vi "Loop_HW.vi"() -> ()   [LabVIEW 2017, in "WCDrive2018.lvlib"]
uses:
  WCDrive2018.lvlib
  Global_SM Out Data.vi
  Global_HW_Status Out.vi
  ProtoType Code/EXAMPLE 2017 competition code/roboRIO Code/Globals/Global_HW_Address_Assignments.vi
  ENUM_ACT_State.ctl
  ENUM_ACT_Action.ctl
  _SHARE ALL/Global Share All/Global_STOP.vi
  <vilib>/Rock Robotics/WPI/MotorControl/WPI_MotorControlType.ctl
  <vilib>/Rock Robotics/SystemInterfaces/DIO/FPGA_DIOPWMChannel.ctl
  <vilib>/Rock Robotics/WPI/PWM/WPI_PWMDeadband.ctl
  <vilib>/Rock Robotics/SystemInterfaces/DIO/FPGA_DIOChannel.ctl
  <vilib>/Rock Robotics/WPI/MotorControl/WPI_MotorControlDeviceRef.ctl
  <vilib>/Rock Robotics/WPI/RobotDrive/WPI_RobotDriveDevRef.ctl
  Enum_HW Cmd Select.ctl
  Cluster_SM to HW Data.ctl
  570cffa0-ccfc-4d94-993e-2857878fdf6e.vi
panel:
  in  "SM CMD Override":bool
  in  "SM_Cmd":T1
  out "Cycle Time (S)":dbl format="%.3g"
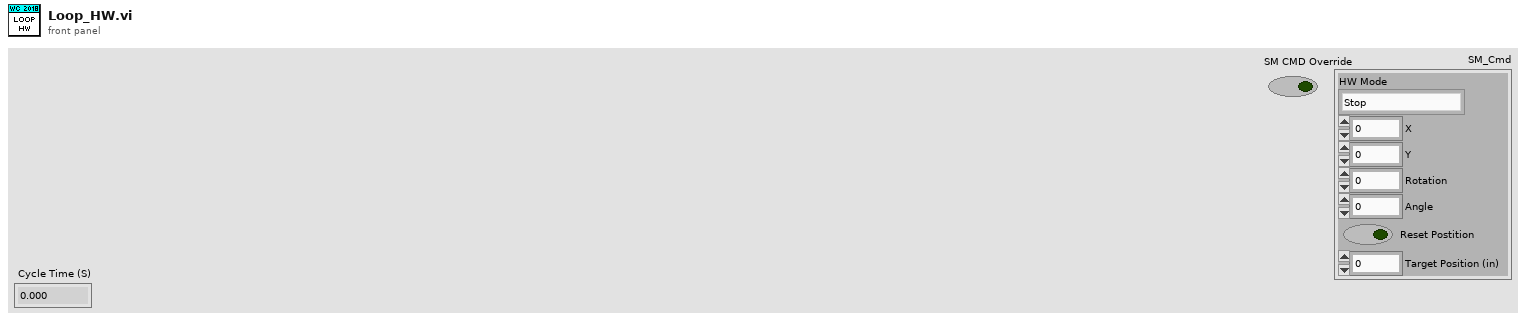
[diagram p1: front panel]
types:
  T1 = typedef "WCDrive2018.lvlib/Cluster_SM to HW Data.ctl" = cluster{"HW Mode":T2, "X":dbl, "Y":dbl, "Rotation":dbl, "Angle":dbl, "Reset Postition":bool, "Target Position (in)":dbl}
  T2 = typedef "WCDrive2018.lvlib/Enum_HW Cmd Select.ctl" = enum16{"Stop", "Vbus", "Positon Lateral", "Postition  FrontBack"}
  T3 = typedef "WPI_RobotDriveDevRef.ctl" = cluster{"DevStatus":errorcluster, "Motors[]":T4[], "Square Inputs":bool, "Max Output":dbl}
  T4 = typedef "WPI_MotorControlDeviceRef.ctl" = cluster{"DeviceStatus":errorcluster, "Type":T5, "PWM":cluster{"PWM Channel":T6, "DeadBand":T7}, "CAN":cluster{"Device Number":u8, "SetOutput VI Ref":variant, "GetOutput VI Ref":variant, "Enable VI Ref":variant, "Disable VI Ref":variant, "Data":variant}, "Invert":bool, "DIO PWM":cluster{"PWM \"Enable\" Channel":T6, "DIOChannel":T8, "PWM Rate":dbl}}
  T5 = typedef "WPI_MotorControlType.ctl" = enum16{"PWM", "CAN", "DIO PWM"}
  T6 = typedef "FPGA_DIOPWMChannel.ctl" = enum8{"PWM 0", "PWM 1", "PWM 2", "PWM 3", "PWM 4", "PWM 5", "PWM 6", "PWM 7", "PWM 8", "PWM 9", "PWM MXP 0", "PWM MXP 1", "PWM MXP 2", "PWM MXP 3", "PWM MXP 4", "PWM MXP 5", "PWM MXP 6", "PWM MXP 7", "PWM MXP 8", "PWM MXP 9", "Invalid"}
  T7 = typedef "WPI_PWMDeadband.ctl" = cluster{"Name":string, "maxPositivePwm":i32, "minPositivePwm":i32, "centerPwm":i32, "maxNegativePwm":i32, "minNegativePwm":i32, "angularRange":u16}
  T8 = typedef "FPGA_DIOChannel.ctl" = enum8{"DIO 0", "DIO 1", "DIO 2", "DIO 3", "DIO 4", "DIO 5", "DIO 6", "DIO 7", "DIO 8", "DIO 9", "DIO MXP 0", "DIO MXP 1", "DIO MXP 2", "DIO MXP 3", "DIO MXP 4", "DIO MXP 5", "DIO MXP 6", "DIO MXP 7", "DIO MXP 8", "DIO MXP 9", "DIO MXP 10", "DIO MXP 11", "DIO MXP 12", "DIO MXP 13", "DIO MXP 14", "DIO MXP 15", "SPI Port CS1", "SPI Port CS2", "SPI Port CS3", "SPI Port MISO", "SPI Port MOSI", "Invalid"}
  T9 = typedef "WCDrive2018.lvlib/ENUM_ACT_State.ctl" = enum16{"_Startup", "_Idle", "_Shutdown"}
  T10 = typedef "WCDrive2018.lvlib/ENUM_ACT_Action.ctl" = enum16{"No Action", "Reset Time", "Reset All", "Initialize SRXs", "_Action B"}
  T11 = typedef "Cluster_WCDrive_SetupData.ctl" = cluster{"Left Master":u8, "Invert Left Master":bool, "Left Slave":u8, "Invert Left Slave":bool, "Right Master":u8, "Invert Right Master":bool, "Right Slave":u8, "Invert Right Slave":bool, "Invert Left Encoder":bool, "Invert Right Encoder":bool}
  T12 = cluster{"State":T9, "Previous State":T9, "Current Time":timestamp, "Previous Time":timestamp, "Start Time":timestamp, "Target Time (ms)":u32, "Cycle Time(S)":dbl, "RobotDriveDevRef":T3, "SM_Cmd":T1, "HW SETUP_WC Drive":T11}
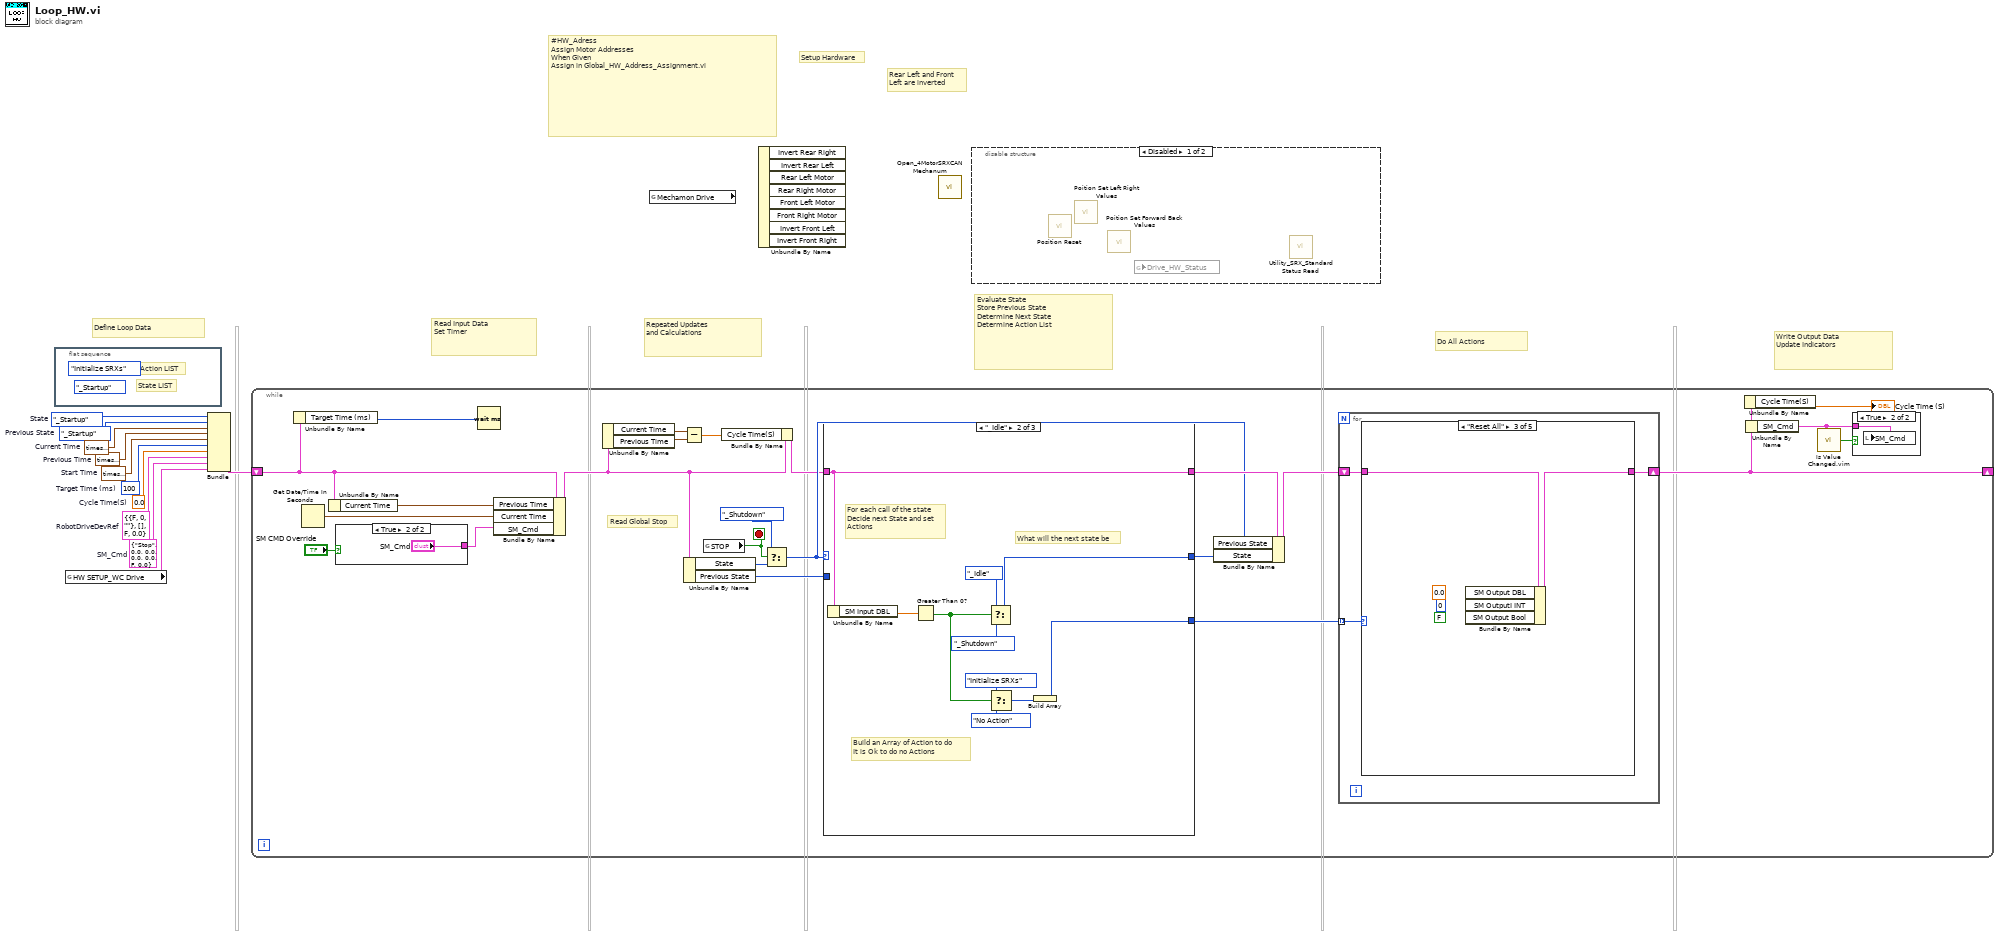
[diagram p0: block diagram]
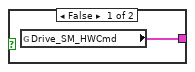
[diagram p2: hidden frame]
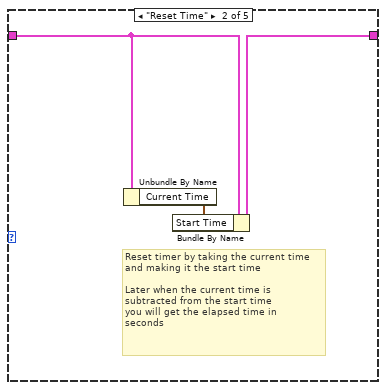
[diagram p5: hidden frame]
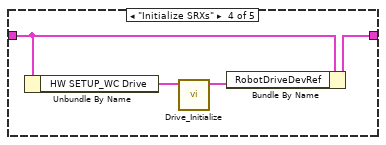
[diagram p6: hidden frame]
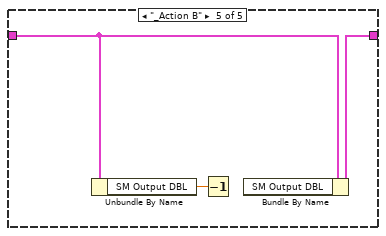
[diagram p7: hidden frame]
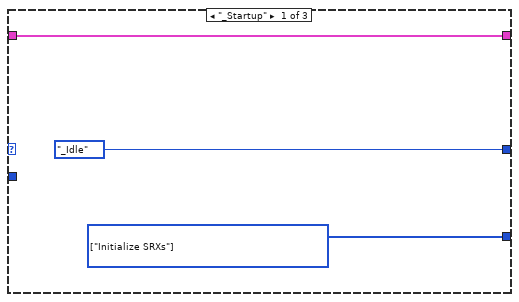
[diagram p8: hidden frame]
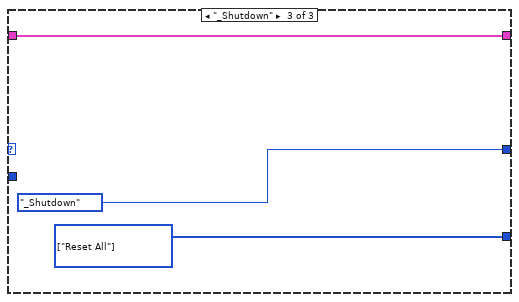
[diagram p9: hidden frame]
diagram:
  w2 = T1 {"HW Mode"=enum."Stop", "X"=0.0, "Y"=0.0, "Rotation"=0.0, "Angle"=0.0, "Reset Postition"=FALSE, "Target Position (in)"=0.0}  # SM_Cmd
  w3 = T3 {"DevStatus"={"status"=FALSE, "code"=0, "source"=""}, "Motors[]"=[], "Square Inputs"=FALSE, "Max Output"=0.0}  # RobotDriveDevRef
  w4 = 0.0  # Cycle Time(S)
  w5 = ENUM_ACT_State."_Startup"  # Previous State
  w6 = timestamp(0 s since 1904-01-01)  # Previous Time
  w7 = u32 100  # Target Time (ms)
  w8 = timestamp(0 s since 1904-01-01)  # Start Time
  w9 = timestamp(0 s since 1904-01-01)  # Current Time
  w10 = ENUM_ACT_State."_Startup"  # State
  # "Define Loop Data"
  # "Repeated Updates\nand Calculations"
  # "Read Input Data\nSet Timer"
  # "Evaluate State\nStore Previous State\nDetermine Next State\nDetermine Action List"
  # "Do All Actions"
  # "Write Output Data\nUpdate Indicators"
  # "#HW_Adress\nAssign Motor Addresses\nWhen Given\nAssign in Global_HW_Address_Assignment.vi"
  # "Rear Left and Front \nLeft are inverted"
  # "Setup Hardware"
  n1 = flat-sequence {
    frame #0 {
      (unwired) ENUM_ACT_State."_Startup" ("State")
      (unwired) ENUM_ACT_Action."Initialize SRXs" ("Action")
      # "State LIST"
      # "Action LIST"
    }
  }
  n2 = global read "Global_HW_Address_Assignments.vi" "HW SETUP_WC Drive"() -> (w1:T11)
  n3 = Bundle("State"=w10, "Previous State"=w5, "Current Time"=w9, "Previous Time"=w6, "Start Time"=w8, "Target Time (ms)"=w7, "Cycle Time(S)"=w4, "RobotDriveDevRef"=w3, "SM_Cmd"=w2, "HW SETUP_WC Drive"=w1) -> (w11:T12)  [unwired: 1 in]
  n4 = while {
    shift-right: [w23] -> _
    shift-left: w11 -> [w26]
    stop <- w31 stop-if-true
    # "Read Global Stop"
    n5 = Unbundle By Name(w26) -> ("Target Time (ms)"=w28:u32)
    n6 = Get Date/Time In Seconds() -> (seconds since 1Jan1904=w35:timestamp)
    n7 = Unbundle By Name(w26) -> ("Current Time"=w27:timestamp)
    n8 = case shown="True" "SM CMD Override" {
      tunnel: [w36 "SM_Cmd"] -> w15
      frame False {
        n9 = global read "Global_SM Out Data.vi" "Drive_SM_HWCmd"() -> (w36:T1)
      }
      frame True {
      }
    }
    n10 = Wait (ms)(milliseconds to wait=w28) -> ()  [unwired: 1 out]
    n11 = Bundle By Name(cluster=w26, "Previous Time"=w27, "Current Time"=w35, "SM_Cmd"=w15) -> (w19:T12)
    n12 = Unbundle By Name(w19) -> ("Current Time"=w20:timestamp, "Previous Time"=w21:timestamp)
    n13 = Subtract(x=w20, y=w21) -> (x-y=w17:dbl)
    n14 = Unbundle By Name(w19) -> ("State"=w29:T9, "Previous State"=w25:T9)
    n15 = global read "Global_STOP.vi" "STOP"() -> (w31:bool)
    n16 = Bundle By Name(cluster=w19, "Cycle Time(S)"=w17) -> (w18:T12)
    n17 = Select(t=ENUM_ACT_State."_Shutdown" ("State"), s=w31, f=w29) -> (s? t:f=w24:T9)
    n18 = case shown="\"_Idle\"" w24 {
      tunnel: w18 -> [w57 w67 w70]
      tunnel: [w57 w67 w70] -> w33
      tunnel: [ENUM_ACT_State."_Idle" ("State") w65 ENUM_ACT_State."_Shutdown" ("State")] -> w32
      tunnel: [w56 w58 w68] -> w16
      tunnel: w25 -> [_ _ _]
      frame "_Startup" {
        w56 = T10[] [enum."Initialize SRXs"] items=["No Action", "Reset Time", "Reset All", "Initialize SRXs", "_Action B"] ("Actions")
      }
      frame "_Idle" {
        # "For each call of the state\nDecide next State and set\nActions"
        # "What will the next state be"
        # "Build an Array of Action to do\nIt is Ok to do no Actions"
        n19 = Unbundle By Name(w67) -> ("SM Input DBL"=w66:dbl)
        n20 = Greater Than 0?(x=w66) -> (x > 0?=w60:bool)
        n21 = Select(t=ENUM_ACT_State."_Idle" ("State"), s=w60, f=ENUM_ACT_State."_Shutdown" ("State")) -> (s? t:f=w65:T9)
        n22 = Select(t=ENUM_ACT_Action."Initialize SRXs" ("Action"), s=w60, f=ENUM_ACT_Action."No Action" ("Action")) -> (s? t:f=w59:T10)
        n23 = Build Array(w59) -> (w58:T10[])
      }
      frame "_Shutdown" {
        w68 = T10[] [enum."Reset All"] items=["No Action", "Reset Time", "Reset All", "Initialize SRXs", "_Action B"] ("Actions")
      }
    }
    n24 = Bundle By Name(cluster=w33, "Previous State"=w24, "State"=w32) -> (w34:T12)
    n25 = for {
      tunnel: w16 -> [w41] mode=indexing
      shift-right: [w40] -> w23
      shift-left: w34 -> [w39]
      n26 = case shown="\"Reset All\"" w41 {
        tunnel: w39 -> [w42 w45 w46 w49 w53]
        tunnel: [w42 w44 w47 w50 w52] -> w40
        frame "No Action" {
        }
        frame "Reset Time" {
          # "Reset timer by taking the current time\nand making it the start time\n\nLater when the current time is \nsubtracted from the start time\nyou will get the elapsed time in \nseconds"
          n27 = Unbundle By Name(w45) -> ("Current Time"=w43:timestamp)
          n28 = Bundle By Name(cluster=w45, "Start Time"=w43) -> (w44:T12)
        }
        frame "Reset All" {
          (unwired) FALSE ("Output Bool")
          (unwired) 0 ("OutputI INT")
          (unwired) 0.0 ("FG Write Value")
          n29 = Bundle By Name(cluster=w46) -> (w47:T12)  [unwired: 3 in]
        }
        frame "Initialize SRXs" {
          n30 = Unbundle By Name(w49) -> ("HW SETUP_WC Drive"=w48:T11)
          n31 = call "Drive_Initialize.vi"("HW SETUP_WC Drive"=w48) -> ("RobotDriveDevRef Out"=w51:T3)  [unwired: 10 in]
          n32 = Bundle By Name(cluster=w49, "RobotDriveDevRef"=w51) -> (w50:T12)
        }
        frame "_Action B" {
          n33 = Unbundle By Name(w53) -> ("SM Output DBL"=w54:dbl)
          n34 = Decrement(x=w54) -> ()  [unwired: 1 out]
          n35 = Bundle By Name(cluster=w53) -> (w52:T12)  [unwired: 1 in]
        }
      }
    }
    n36 = Unbundle By Name(w23) -> ("Cycle Time(S)"=→"Cycle Time (S)":dbl)
    n37 = Unbundle By Name(w23) -> ("SM_Cmd"=w13:T1)
    n38 = call "Is Value Changed.vim"("value"=w13) -> ("changed or first call?"=w14:bool)
    n39 = case shown="True" w14 {
      tunnel: w13 -> [_ w38]
      frame False {
      }
      frame True {
        n40 = local write "SM_Cmd"(w38) -> ()
      }
    }
  }
  n41 = global read "Global_HW_Address_Assignments.vi" "Mechamon Drive"() -> ()  [unwired: 1 out]
  n42 = Unbundle By Name() -> ()  [unwired: 1 in, 8 out]
  n43 = call "Open_4MotorSRXCAN Mechanum.vi"() -> ()  [unwired: 14 in, 2 out]
  n44 = disable-structure shown="Disabled" {
    frame Disabled {
      n45 = call "Position Reset.vi"() -> ()  [unwired: 10 in, 2 out]
      n46 = call "Poition Set Left Right Values.vi"() -> ()  [unwired: 10 in, 2 out]
      n47 = call "Poition Set Forward Back Values.vi"() -> ()  [unwired: 10 in, 2 out]
      n48 = global read "Global_HW_Status Out.vi" "Drive_HW_Status"() -> ()  [unwired: 1 in]
      n49 = call "Utility_SRX_Standard Status Read.vi"() -> ()  [unwired: 9 in, 3 out]
    }
    frame Enabled {
    }
  }
